vi "Encoders.vi"(3 "Reset All":bool) -> (0 "Avg Absolute Rate":dbl, 1 "Avg Absolute Distance":dbl)   [LabVIEW 2016]
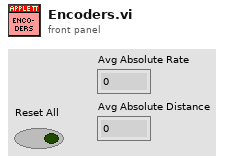
[diagram p1: front panel]
types:
  T1 = typedef "WPI_EncoderDevRef.ctl" = cluster{"DevStatus":errorcluster, "EncoderIndex":T2, "CounterIndex":T3, "DistancePerCount":dbl, "Decoding Type":T4}
  T2 = typedef "FPGA_EncoderIdx.ctl" = enum8{"Enc 0", "Enc 1", "Enc 2", "Enc 3", "Enc 4", "Enc 5", "Enc 6", "Enc 7", "Invalid"}
  T3 = typedef "FPGA_CounterCtrSystemIndex.ctl" = enum8{"Ctr 0", "Ctr 1", "Ctr 2", "Ctr 3", "Ctr 4", "Ctr 5", "Ctr 6", "Ctr 7", "Invalid"}
  T4 = typedef "WPI_EncoderType.ctl" = enum16{"1x", "2x", "4x"}
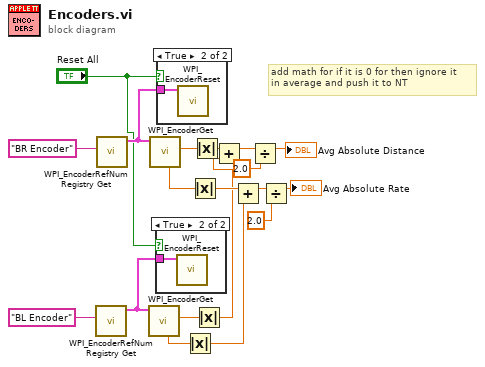
[diagram p0: block diagram]
diagram:
  # "add math for if it is 0 for then ignore it \nin average and push it to NT"
  n1 = call <vilib>:"WPI_EncoderRefNum Registry Get.vi"("refnum name"="BL Encoder") -> ("EncoderDevRef"=w12:T1)  [unwired: 9 in, 1 out]
  n2 = call <vilib>:"WPI_EncoderRefNum Registry Get.vi"("refnum name"="BR Encoder") -> ("EncoderDevRef"=w18:T1)  [unwired: 9 in, 1 out]
  n3 = call <vilib>:"WPI_EncoderGet.vi"("EncoderDevRef"=w12) -> ("Distance"=w9:dbl, "Rate"=w5:dbl)  [unwired: 5 in, 4 out]
  n4 = call <vilib>:"WPI_EncoderGet.vi"("EncoderDevRef"=w18) -> ("Distance"=w16:dbl, "Rate"=w17:dbl)  [unwired: 5 in, 4 out]
  n5 = case shown="True" "Reset All" {
    tunnel: w12 -> [_ w20]
    frame False {
    }
    frame True {
      n6 = call <vilib>:"WPI_EncoderReset.vi"("EncoderDevRef"=w20) -> ()  [unwired: 9 in, 2 out]
    }
  }
  n7 = case shown="True" "Reset All" {
    tunnel: w18 -> [_ w21]
    frame False {
    }
    frame True {
      n8 = call <vilib>:"WPI_EncoderReset.vi"("EncoderDevRef"=w21) -> ()  [unwired: 9 in, 2 out]
    }
  }
  n9 = Absolute Value(x=w5) -> (abs(x)=w1:dbl)
  n10 = Absolute Value(x=w17) -> (abs(x)=w14:dbl)
  n11 = Absolute Value(x=w16) -> (abs(x)=w15:dbl)
  n12 = Absolute Value(x=w9) -> (abs(x)=w2:dbl)
  n13 = Add(x=w15, y=w2) -> (x+y=w10:dbl)
  n14 = Add(x=w14, y=w1) -> (x+y=w6:dbl)
  n15 = Divide(x=w10, y=2.0) -> (x/y=→"Avg Absolute Distance":dbl)
  n16 = Divide(x=w6, y=2.0) -> (x/y=→"Avg Absolute Rate":dbl)
